vi "build intensity array.vi"(8 "error in":errorcluster, 11 "display array in":T2(array[cluster])=[{"X name"="", "Y name "="", "counts"=0.0, "gate 1"=[], "count rate"=0.0, "X Peak"=0.0, "Y Peak"=0.0, "cathode position"=0.0}, {"X name"="", "Y name "="", "counts"=0.0, "gate 1"=[], "count rate"=0.0, "X Peak"=0.0, "Y Peak"=0.0, "cathode position"=0.0}, {"X name"="", "Y name "="", "counts"=0.0, "gate 1"=[], "count rate"=0.0, "X Peak"=0.0, "Y Peak"=0.0, "cathode position"=0.0}, {"X name"="", "Y name "="", "counts"=0.0, "gate 1"=[], "count rate"=0.0, "X Peak"=0.0, "Y Peak"=0.0, "cathode position"=0.0}, {"X name"="1", "Y name "="", "counts"=0.0, "gate 1"=[], "count rate"=0.0, "X Peak"=0.0, "Y Peak"=0.0, "cathode position"=0.0}]) -> (0 "error out":errorcluster, 3 "display array out":T2(array[cluster]))   [LabVIEW 2016]
doc: "creates memory space for intensity plots to be displayed on realtime data aquire vi"
panel:
  in  "xy position cluster":T1
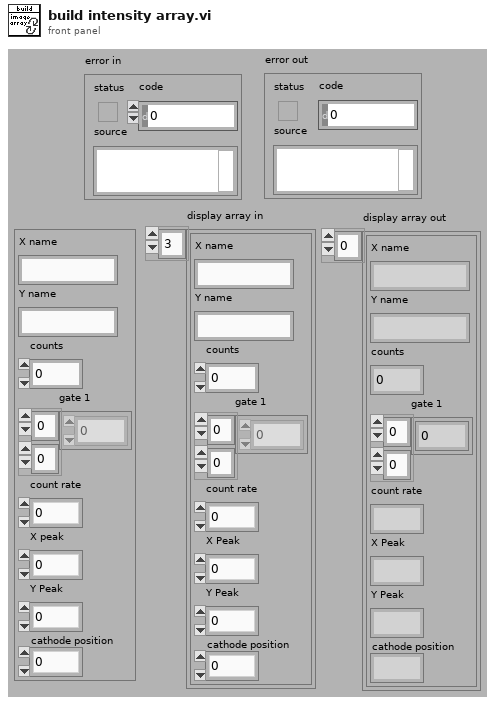
[diagram p1: front panel]
types:
  T1 = cluster{"X name":string, "Y name ":string, "counts":dbl, "gate 1":dbl[][], "count rate":dbl, "X peak":dbl, "Y Peak":dbl, "cathode position":dbl}
  T2 = cluster{"X name":string, "Y name ":string, "counts":dbl, "gate 1":dbl[][], "count rate":dbl, "X Peak":dbl, "Y Peak":dbl, "cathode position":dbl}[]
  T3 = cluster{"X name":string, "Y name ":string, "counts":dbl, "gate 1":dbl[][], "count rate":dbl, "X Peak":dbl, "Y Peak":dbl, "cathode position":dbl}
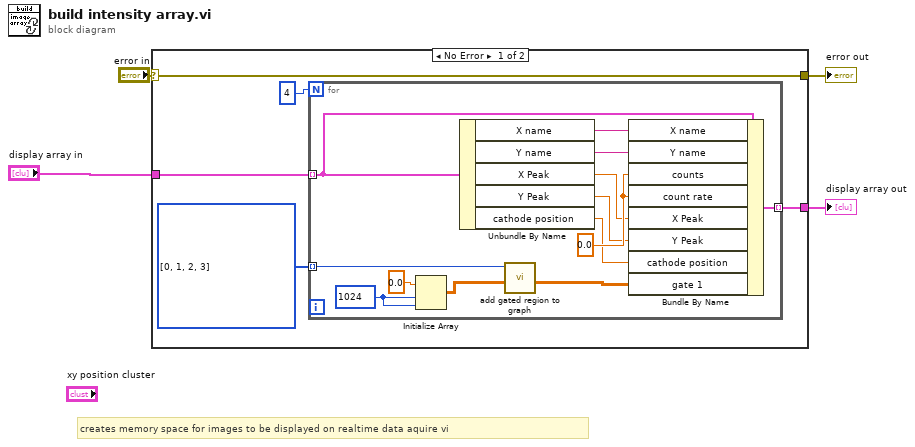
[diagram p0: block diagram]
diagram:
  # "creates memory space for images to be displayed on realtime data aquire vi"
  n1 = case shown="No Error" "error in" {
    selector: "error in" -> [w7 w24]
    tunnel: [w7 w24] -> w3
    tunnel: [w9 w23] -> w2
    tunnel: "display array in" -> [w8 w23]
    frame No Error {
      w6 = u16[] [0, 1, 2, 3] items=["pulser", "gate 1", "gate 2", "gate 3", "none"]
      n2 = for {
        N: 4 -> [_]
        tunnel: w8 -> [w21] mode=indexing
        tunnel: [w22] -> w9 mode=indexing
        tunnel: w6 -> [w14] mode=indexing
        w10 = 1024 ("X Resolution")
        w18 = 0.0 ("counts")
        n3 = Initialize Array(0.0 ("element"), w10, w10) -> (w11:dbl[][])
        n4 = Unbundle By Name(w21) -> ("X name"=w20:string, "Y name"=w19:string, "X Peak"=w16:dbl, "Y Peak"=w17:dbl, "cathode position"=w15:dbl)
        n5 = call "add gated region to graph.vi"("image in"=w11, "which gate"=w14) -> ("image out"=w13:dbl[][])  [unwired: 7 in, 2 out]
        n6 = Bundle By Name(cluster=w21, "X name"=w20, "Y name"=w19, "counts"=w18, "count rate"=w18, "X Peak"=w16, "Y Peak"=w17, "cathode position"=w15, "gate 1"=w13) -> (w22:T3)
      }
    }
    frame Error {
    }
  }
  "error out" <- w3
  "display array out" <- w2
